vi "StaticCalibration.vi"(0 "SENSOR":T1, 11 "error in (no error)":errorcluster caption="错误输入（无错误）") -> (4 "Vres":dbl, 6 "Angle out":dbl, 8 "Vres_FD":i32, 10 "OK？":bool, 15 "error out":errorcluster caption="错误输出")   [LabVIEW 2020]
doc: "该模板用于创建子VI。"
uses:
  Global_Variable/Global.vi
panel:
  out "T2(%)":dbl
  out "T1(%)":dbl
  out "S(%)":dbl
  out "P(%)":dbl
  out "T2ROC_1+T2ROC_2":i32
  out "T1ROC_1+T1ROC_2":i32
  out "PROC_1":i32
  out "T2ROC_1":i32
  out "T1ROC_1":i32
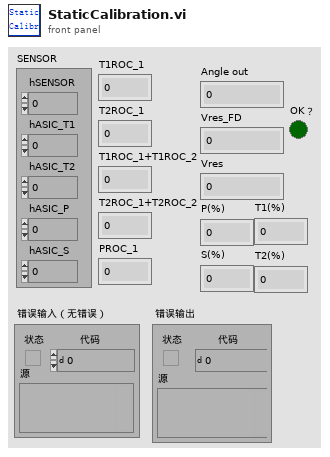
[diagram p1: front panel]
types:
  T1 = cluster{"hSENSOR":i32, "hASIC_T1":i32, "hASIC_T2":i32, "hASIC_P":i32, "hASIC_S":i32}
  T2 = cluster{"主信号":cluster{"单位":string, "下限":dbl, "上限":dbl}, "副信号":cluster{"单位":string, "下限":dbl, "上限":dbl}, "主副和":cluster{"单位":string, "下限":dbl, "上限":dbl}, "主副差":cluster{"单位":string, "下限":dbl, "上限":dbl}, "Vres":cluster{"单位":string, "下限":dbl, "上限":dbl}}
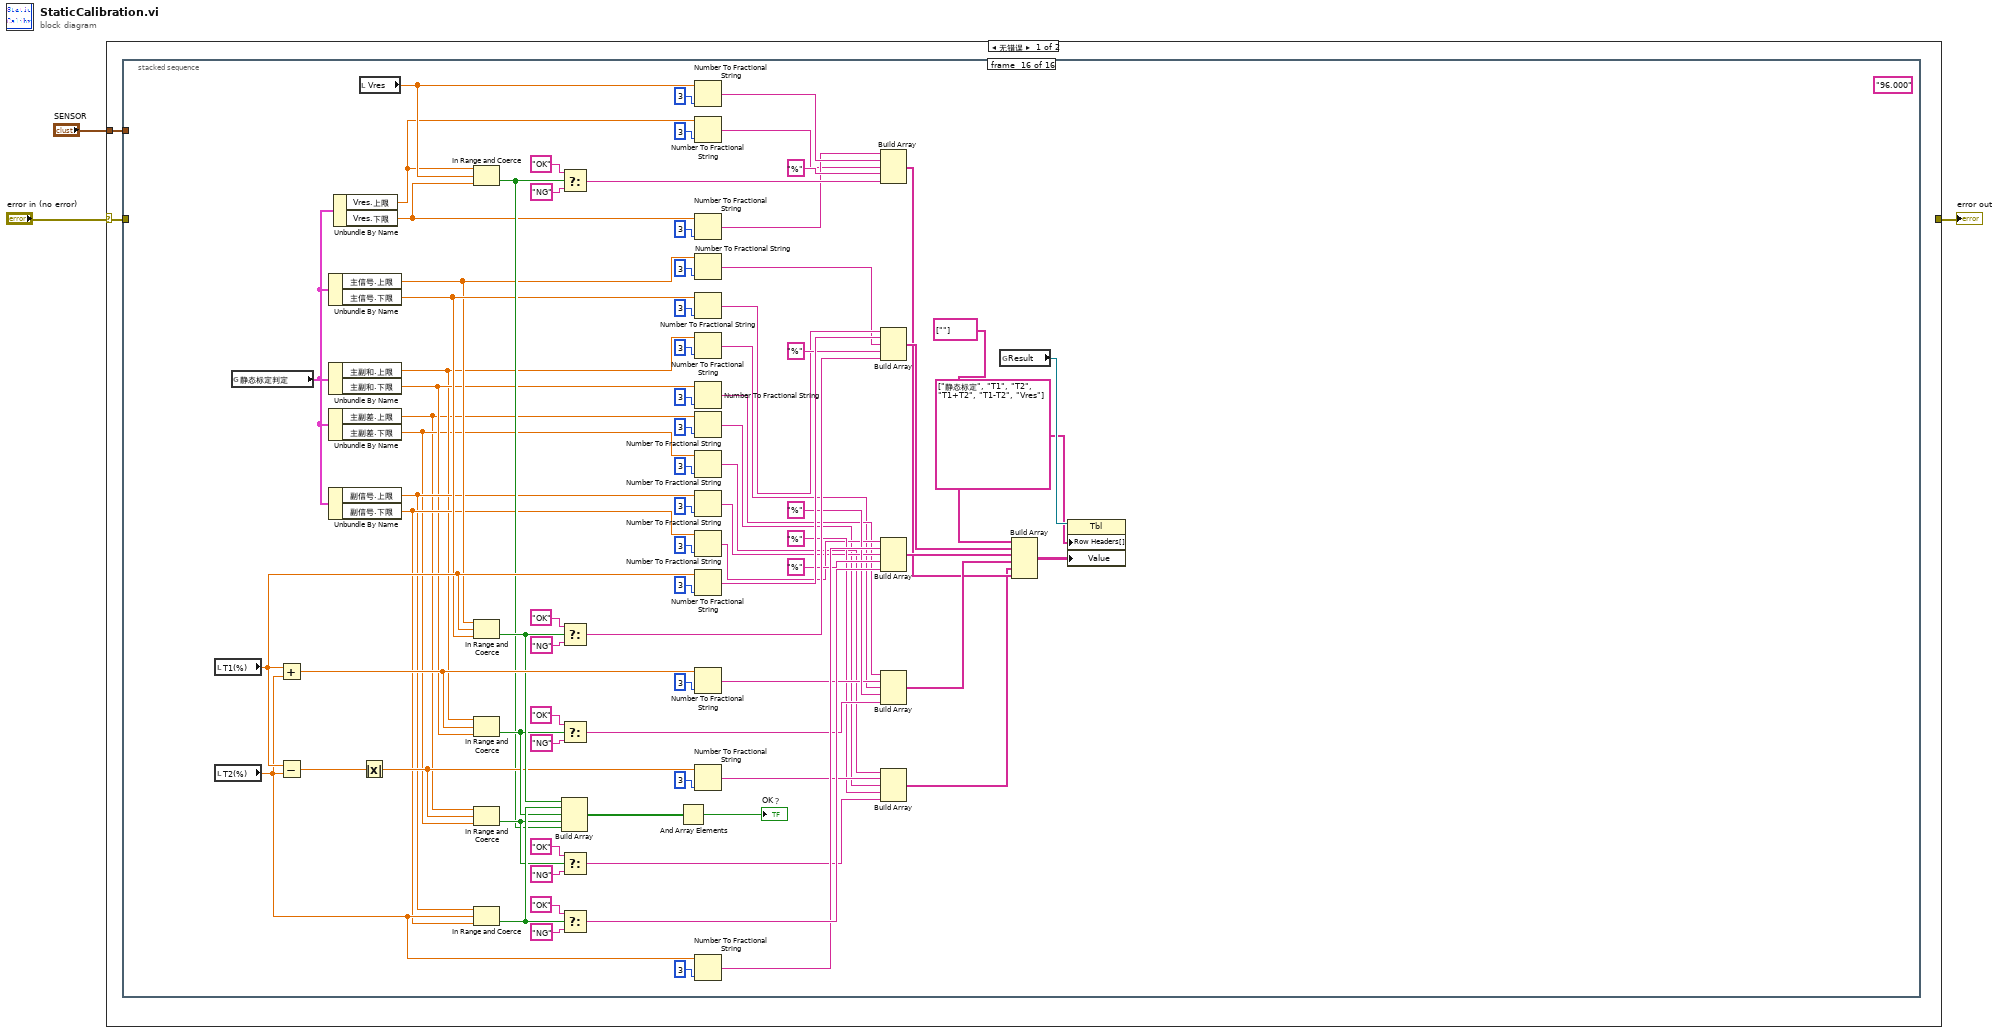
[diagram p0: block diagram]
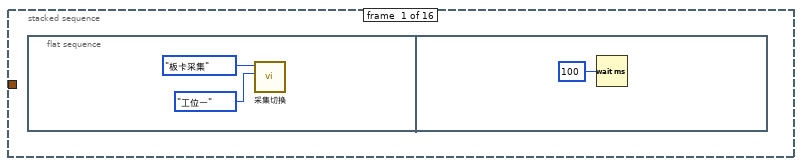
[diagram p2: hidden frame]
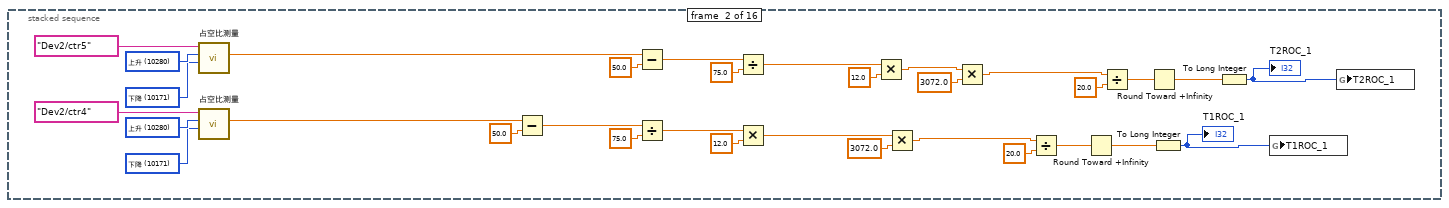
[diagram p3: hidden frame]
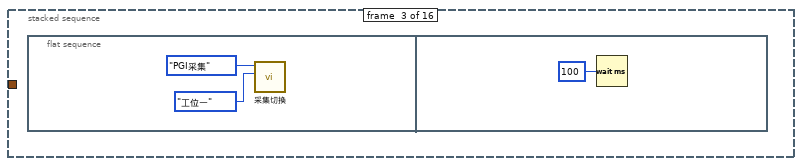
[diagram p4: hidden frame]
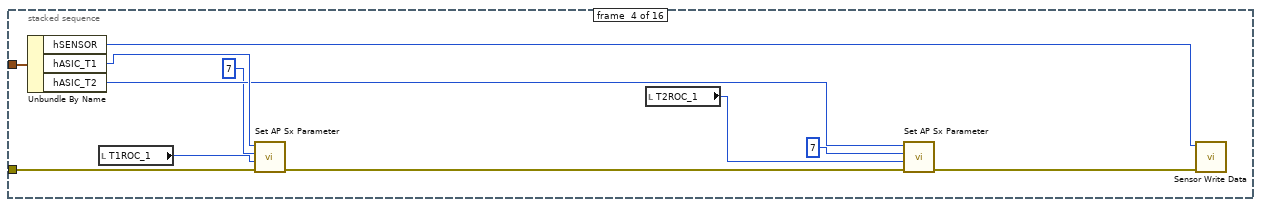
[diagram p5: hidden frame]
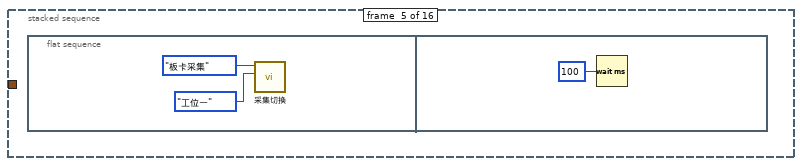
[diagram p6: hidden frame]
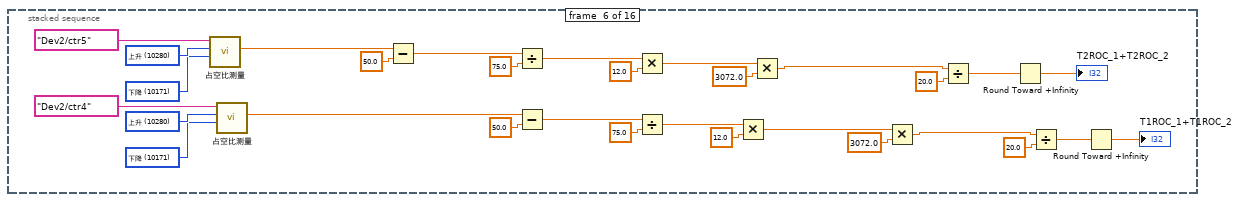
[diagram p7: hidden frame]
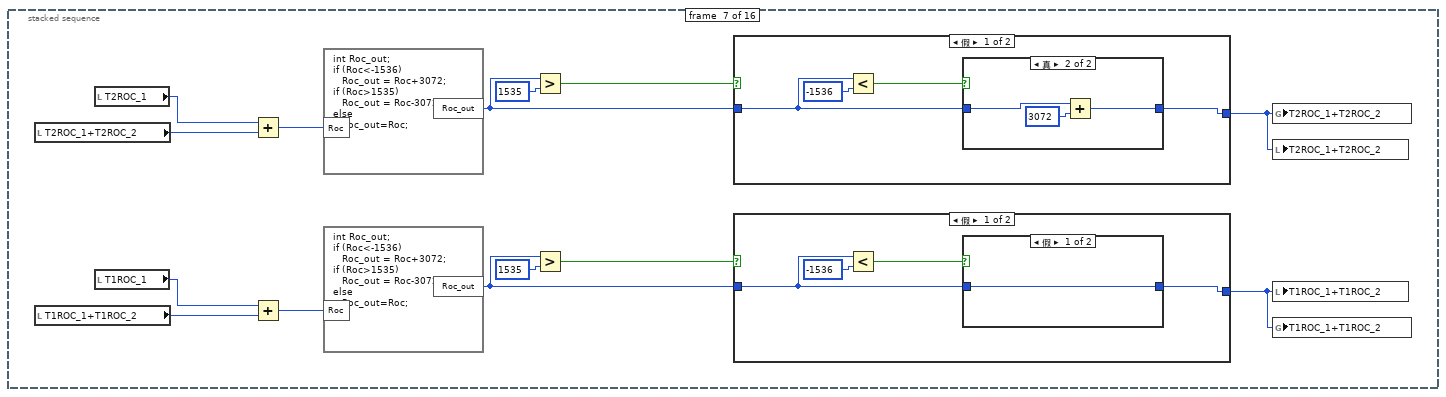
[diagram p8: hidden frame]
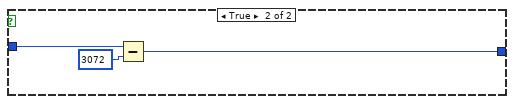
[diagram p10: hidden frame]
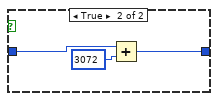
[diagram p11: hidden frame]
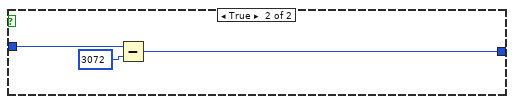
[diagram p12: hidden frame]
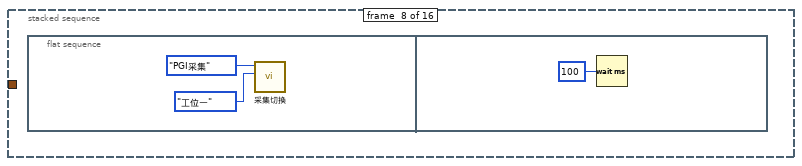
[diagram p13: hidden frame]
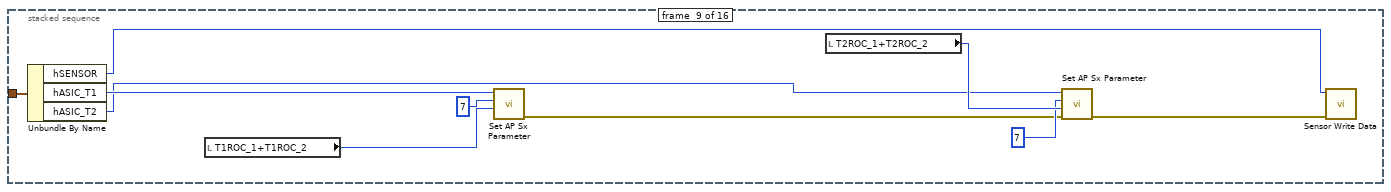
[diagram p14: hidden frame]
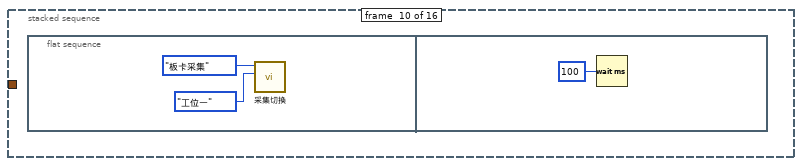
[diagram p15: hidden frame]
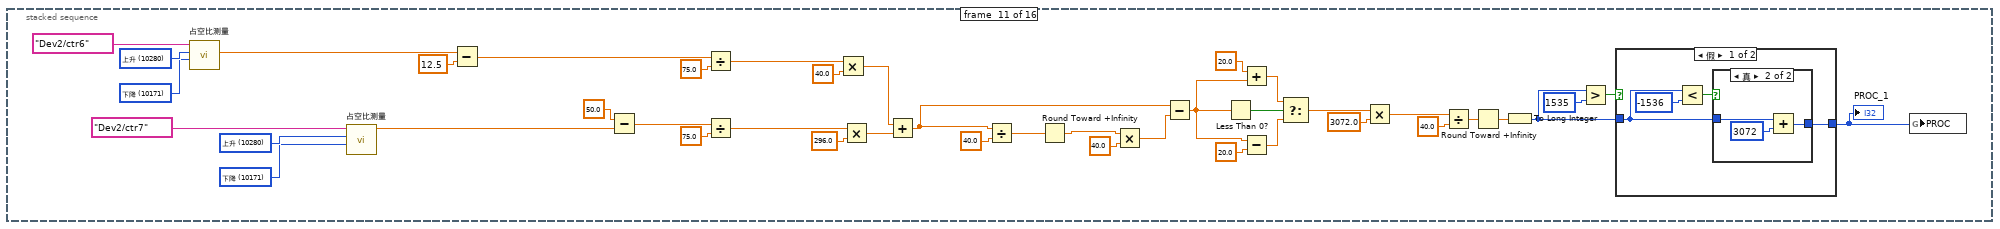
[diagram p16: hidden frame]
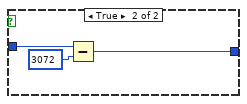
[diagram p18: hidden frame]
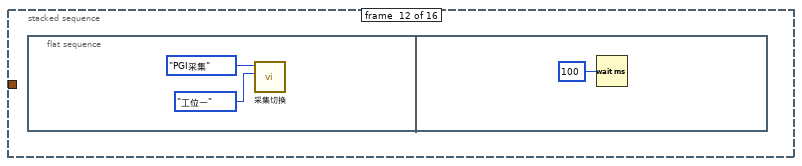
[diagram p19: hidden frame]
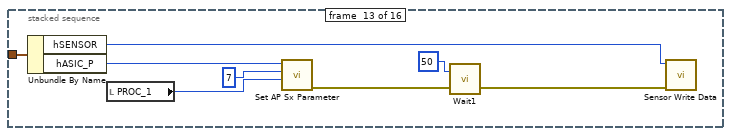
[diagram p20: hidden frame]
diagram:
  n1 = case shown="无错误" "error in (no error)" {
    selector: "error in (no error)" -> [w4 w309]
    tunnel: [_ w309] -> w2
    tunnel: "SENSOR" -> [w5 _]
    frame No Error {
      n2 = stacked-sequence {
        tunnel: w5 -> [_ _ _ w52 _ _ _ _ w135 _ _ _ w198 _ _ _]
        tunnel: w4 -> [_ _ _ w44 _ _ _ _ _ _ _ _ _ _ _ _]
        frame #0 {
          n3 = flat-sequence {
            frame #0 {
              n4 = call "采集切换.vi"("工位"=enum16{"工位一", "工位二"}."工位一", "采集方式"=enum16{"板卡采集", "PGI采集"}."板卡采集") -> ()  [unwired: 10 in]
            }
            frame #1 {
              n5 = Wait (ms)(milliseconds to wait=u32 100 ("等待时间（毫秒）")) -> ()  [unwired: 1 out]
            }
          }
        }
        frame #1 {
          w9 = 10171 items=["上升"=10280, "下降"=10171] ("starting edge2")
          w10 = 10280 items=["上升"=10280, "下降"=10171] ("starting edge1")
          w11 = 10171 items=["上升"=10280, "下降"=10171] ("starting edge2")
          w12 = 10280 items=["上升"=10280, "下降"=10171] ("starting edge1")
          n6 = call "占空比测量.vi"("计数器"=tag "Dev2/ctr5" ("counter"), "starting edge1"=w10, "starting edge2"=w9) -> ("占空比2(%)"=w13:dbl)  [unwired: 4 in, 3 out]
          n7 = call "占空比测量.vi"("计数器"=tag "Dev2/ctr4" ("counter"), "starting edge1"=w12, "starting edge2"=w11) -> ("占空比2(%)"=w16:dbl)  [unwired: 4 in, 3 out]
          n8 = Subtract(x=w16, y=50.0) -> (x-y=w39:dbl)
          n9 = Subtract(x=w13, y=50.0) -> (x-y=w24:dbl)
          n10 = Divide(x=w39, y=75.0) -> (x/y=w37:dbl)
          n11 = Divide(x=w24, y=75.0) -> (x/y=w26:dbl)
          n12 = Multiply(x=w37, y=12.0) -> (x*y=w35:dbl)
          n13 = Multiply(x=w26, y=12.0) -> (x*y=w28:dbl)
          n14 = Multiply(x=w35, y=3072.0) -> (x*y=w33:dbl)
          n15 = Multiply(x=w28, y=3072.0) -> (x*y=w30:dbl)
          n16 = Divide(x=w33, y=20.0) -> (x/y=w20:dbl)
          n17 = Round Toward +Infinity(x=w20) -> (ceil(x): smallest int >= x=w18:dbl)
          n18 = Divide(x=w30, y=20.0) -> (x/y=w19:dbl)
          n19 = Round Toward +Infinity(x=w19) -> (ceil(x): smallest int >= x=w17:dbl)
          n20 = To Long Integer(number=w18) -> (32bit integer=w14:i32)
          "T1ROC_1" <- w14
          n21 = To Long Integer(number=w17) -> (32bit integer=w15:i32)
          "T2ROC_1" <- w15
          n22 = global write "Global.vi" "T1ROC_1"(w14) -> ()
          n23 = global write "Global.vi" "T2ROC_1"(w15) -> ()
        }
        frame #2 {
          n24 = flat-sequence {
            frame #0 {
              n25 = call "采集切换.vi"("工位"=enum16{"工位一", "工位二"}."工位一", "采集方式"=enum16{"板卡采集", "PGI采集"}."PGI采集") -> ()  [unwired: 10 in]
            }
            frame #1 {
              n26 = Wait (ms)(milliseconds to wait=u32 100 ("等待时间（毫秒）")) -> ()  [unwired: 1 out]
            }
          }
        }
        frame #3 {
          n27 = Unbundle By Name(w52) -> ("hSENSOR"=w49:i32, "hASIC_T1"=w51:i32, "hASIC_T2"=w50:i32)
          n28 = local read "T1ROC_1"() -> (w53:i32)
          n29 = call "Set AP Sx Parameter.vi"("error in (no error)"=w44, "para2"=w53, "asicBitsName"=7, "asicHandle"=w51) -> ("error out"=w46:errorcluster)  [unwired: 6 in, 1 out]
          n30 = local read "T2ROC_1"() -> (w54:i32)
          n31 = call "Set AP Sx Parameter.vi"("error in (no error)"=w46, "para2"=w54, "asicBitsName"=7, "asicHandle"=w50) -> ("error out"=w45:errorcluster)  [unwired: 6 in, 1 out]
          n32 = call "Sensor Write Data.vi"("error in (no error)"=w45, "sensorHandle"=w49) -> ()  [unwired: 8 in, 2 out]
        }
        frame #4 {
          n33 = flat-sequence {
            frame #0 {
              n34 = call "采集切换.vi"("工位"=enum16{"工位一", "工位二"}."工位一", "采集方式"=enum16{"板卡采集", "PGI采集"}."板卡采集") -> ()  [unwired: 10 in]
            }
            frame #1 {
              n35 = Wait (ms)(milliseconds to wait=u32 100 ("等待时间（毫秒）")) -> ()  [unwired: 1 out]
            }
          }
        }
        frame #5 {
          w58 = 10171 items=["上升"=10280, "下降"=10171] ("starting edge2")
          w59 = 10280 items=["上升"=10280, "下降"=10171] ("starting edge1")
          w60 = 10171 items=["上升"=10280, "下降"=10171] ("starting edge2")
          w61 = 10280 items=["上升"=10280, "下降"=10171] ("starting edge1")
          n36 = call "占空比测量.vi"("计数器"=tag "Dev2/ctr5", "starting edge1"=w59, "starting edge2"=w58) -> ("占空比2(%)"=w65:dbl)  [unwired: 4 in, 3 out]
          n37 = call "占空比测量.vi"("计数器"=tag "Dev2/ctr4", "starting edge1"=w61, "starting edge2"=w60) -> ("占空比2(%)"=w62:dbl)  [unwired: 4 in, 3 out]
          n38 = Subtract(x=w65, y=50.0) -> (x-y=w87:dbl)
          n39 = Divide(x=w87, y=75.0) -> (x/y=w86:dbl)
          n40 = Subtract(x=w62, y=50.0) -> (x-y=w80:dbl)
          n41 = Multiply(x=w86, y=12.0) -> (x*y=w85:dbl)
          n42 = Divide(x=w80, y=75.0) -> (x/y=w81:dbl)
          n43 = Multiply(x=w81, y=12.0) -> (x*y=w82:dbl)
          n44 = Multiply(x=w85, y=3072.0) -> (x*y=w84:dbl)
          n45 = Multiply(x=w82, y=3072.0) -> (x*y=w83:dbl)
          n46 = Divide(x=w84, y=20.0) -> (x/y=w78:dbl)
          n47 = Round Toward +Infinity(x=w78) -> (ceil(x): smallest int >= x=→"T2ROC_1+T2ROC_2":dbl)
          n48 = Divide(x=w83, y=20.0) -> (x/y=w79:dbl)
          n49 = Round Toward +Infinity(x=w79) -> (ceil(x): smallest int >= x=→"T1ROC_1+T1ROC_2":dbl)
        }
        frame #6 {
          n50 = local read "T2ROC_1+T2ROC_2"() -> (w90:i32)
          n51 = local read "T1ROC_1+T1ROC_2"() -> (w91:i32)
          n52 = local read "T2ROC_1"() -> (w98:i32)
          n53 = local read "T1ROC_1"() -> (w99:i32)
          n54 = Add(x=w98, y=w90) -> (x+y=w100:i32)
          n55 = Add(x=w99, y=w91) -> (x+y=w101:i32)
          n56 = formula code="int Roc_out;\nif (Roc<-1536)\n   Roc_out = Roc+3072;\nif (Roc>1535)\n   Roc_out = Roc-3072;\nelse\n   Roc_out=Roc;"("Roc"=w100) -> ("Roc_out"=w92:i32)
          n57 = formula code="int Roc_out;\nif (Roc<-1536)\n   Roc_out = Roc+3072;\nif (Roc>1535)\n   Roc_out = Roc-3072;\nelse\n   Roc_out=Roc;"("Roc"=w101) -> ("Roc_out"=w95:i32)
          n58 = Greater?(x=w92, y=1535) -> (0:w93:bool)
          n59 = Greater?(x=w95, y=1535) -> (0:w96:bool)
          n60 = case shown="假" w93 {
            tunnel: w92 -> [w103 w111]
            tunnel: [w102 w110] -> w88
            frame False {
              n61 = Less?(x=w103, y=-1536) -> (x < y?=w104:bool)
              n62 = case shown="真" w104 {
                tunnel: w103 -> [w106 w109]
                tunnel: [w106 w107] -> w102
                frame False {
                }
                frame True {
                  n63 = Add(x=w109, y=3072) -> (x+y=w107:i32)
                }
              }
            }
            frame True {
              n64 = Subtract(x=w111, y=3072) -> (x-y=w110:i32)
            }
          }
          n65 = case shown="假" w96 {
            tunnel: w95 -> [w114 w122]
            tunnel: [w113 w121] -> w89
            frame False {
              n66 = Less?(x=w114, y=-1536) -> (x < y?=w115:bool)
              n67 = case shown="假" w115 {
                tunnel: w114 -> [w117 w120]
                tunnel: [w117 w118] -> w113
                frame False {
                }
                frame True {
                  n68 = Add(x=w120, y=3072) -> (x+y=w118:i32)
                }
              }
            }
            frame True {
              n69 = Subtract(x=w122, y=3072) -> (x-y=w121:i32)
            }
          }
          n70 = global write "Global.vi" "T2ROC_1+T2ROC_2"(w88) -> ()
          n71 = local write "T2ROC_1+T2ROC_2"(w88) -> ()
          n72 = local write "T1ROC_1+T1ROC_2"(w89) -> ()
          n73 = global write "Global.vi" "T1ROC_1+T1ROC_2"(w89) -> ()
        }
        frame #7 {
          n74 = flat-sequence {
            frame #0 {
              n75 = call "采集切换.vi"("工位"=enum16{"工位一", "工位二"}."工位一", "采集方式"=enum16{"板卡采集", "PGI采集"}."PGI采集") -> ()  [unwired: 10 in]
            }
            frame #1 {
              n76 = Wait (ms)(milliseconds to wait=u32 100 ("等待时间（毫秒）")) -> ()  [unwired: 1 out]
            }
          }
        }
        frame #8 {
          n77 = Unbundle By Name(w135) -> ("hSENSOR"=w132:i32, "hASIC_T1"=w134:i32, "hASIC_T2"=w133:i32)
          n78 = local read "T1ROC_1+T1ROC_2"() -> (w131:i32)
          n79 = call "Set AP Sx Parameter.vi"("para2"=w131, "asicBitsName"=7, "asicHandle"=w134) -> ("error out"=w128:errorcluster)  [unwired: 7 in, 1 out]
          n80 = local read "T2ROC_1+T2ROC_2"() -> (w136:i32)
          n81 = call "Set AP Sx Parameter.vi"("error in (no error)"=w128, "para2"=w136, "asicBitsName"=7, "asicHandle"=w133) -> ("error out"=w127:errorcluster)  [unwired: 6 in, 1 out]
          n82 = call "Sensor Write Data.vi"("error in (no error)"=w127, "sensorHandle"=w132) -> ()  [unwired: 8 in, 2 out]
        }
        frame #9 {
          n83 = flat-sequence {
            frame #0 {
              n84 = call "采集切换.vi"("工位"=enum16{"工位一", "工位二"}."工位一", "采集方式"=enum16{"板卡采集", "PGI采集"}."板卡采集") -> ()  [unwired: 10 in]
            }
            frame #1 {
              n85 = Wait (ms)(milliseconds to wait=u32 100 ("等待时间（毫秒）")) -> ()  [unwired: 1 out]
            }
          }
        }
        frame #10 {
          w140 = 10171 items=["上升"=10280, "下降"=10171] ("starting edge2")
          w141 = 10280 items=["上升"=10280, "下降"=10171] ("starting edge1")
          w142 = 10171 items=["上升"=10280, "下降"=10171] ("starting edge2")
          w143 = 10280 items=["上升"=10280, "下降"=10171] ("starting edge1")
          n86 = call "占空比测量.vi"("计数器"=tag "Dev2/ctr6", "starting edge1"=w143, "starting edge2"=w142) -> ("占空比2(%)"=w148:dbl)  [unwired: 4 in, 3 out]
          n87 = call "占空比测量.vi"("计数器"=tag "Dev2/ctr7", "starting edge1"=w141, "starting edge2"=w140) -> ("占空比(%)"=w147:dbl)  [unwired: 4 in, 3 out]
          n88 = Subtract(x=w148, y=12.5) -> (x-y=w180:dbl)
          n89 = Subtract(x=50.0, y=w147) -> (x-y=w174:dbl)
          n90 = Divide(x=w180, y=75.0) -> (x/y=w178:dbl)
          n91 = Divide(x=w174, y=75.0) -> (x/y=w172:dbl)
          n92 = Multiply(x=w178, y=40.0) -> (x*y=w176:dbl)
          n93 = Multiply(x=w172, y=296.0) -> (x*y=w170:dbl)
          n94 = Add(x=w176, y=w170) -> (x+y=w164:dbl)
          n95 = Divide(x=w164, y=40.0) -> (x/y=w168:dbl)
          n96 = Round Toward +Infinity(x=w168) -> (ceil(x): smallest int >= x=w166:dbl)
          n97 = Multiply(x=w166, y=40.0) -> (x*y=w165:dbl)
          n98 = Subtract(x=w164, y=w165) -> (x-y=w160:dbl)
          n99 = Less Than 0?(x=w160) -> (x < 0?=w159:bool)
          n100 = Add(x=20.0, y=w160) -> (x+y=w162:dbl)
          n101 = Subtract(x=w160, y=20.0 ("x")) -> (x-y=w158:dbl)
          n102 = Select(t=w162, s=w159, f=w158) -> (s? t:f=w157:dbl)
          n103 = Multiply(x=w157, y=3072.0) -> (x*y=w155:dbl)
          n104 = Divide(x=w155, y=40.0) -> (x/y=w150:dbl)
          n105 = Round Toward +Infinity(x=w150) -> (ceil(x): smallest int >= x=w149:dbl)
          n106 = To Long Integer(number=w149) -> (32bit integer=w153:i32)
          n107 = Greater?(x=w153, y=1535) -> (0:w151:bool)
          n108 = case shown="假" w151 {
            tunnel: w153 -> [w183 w191]
            tunnel: [w182 w190] -> w144
            frame False {
              n109 = Less?(x=w183, y=-1536) -> (x < y?=w184:bool)
              n110 = case shown="真" w184 {
                tunnel: w183 -> [w186 w189]
                tunnel: [w186 w187] -> w182
                frame False {
                }
                frame True {
                  n111 = Add(x=w189, y=3072) -> (x+y=w187:i32)
                }
              }
            }
            frame True {
              n112 = Subtract(x=w191, y=3072) -> (x-y=w190:i32)
            }
          }
          "PROC_1" <- w144
          n113 = global write "Global.vi" "PROC"(w144) -> ()
        }
        frame #11 {
          n114 = flat-sequence {
            frame #0 {
              n115 = call "采集切换.vi"("工位"=enum16{"工位一", "工位二"}."工位一", "采集方式"=enum16{"板卡采集", "PGI采集"}."PGI采集") -> ()  [unwired: 10 in]
            }
            frame #1 {
              n116 = Wait (ms)(milliseconds to wait=u32 100 ("等待时间（毫秒）")) -> ()  [unwired: 1 out]
            }
          }
        }
        frame #12 {
          n117 = Unbundle By Name(w198) -> ("hSENSOR"=w197:i32, "hASIC_P"=w196:i32)
          n118 = local read "PROC_1"() -> (w201:i32)
          n119 = call "Set AP Sx Parameter.vi"("para2"=w201, "asicBitsName"=7, "asicHandle"=w196) -> ("error out"=w203:errorcluster)  [unwired: 7 in, 1 out]
          n120 = call "Wait1.vi"("error in (no error)"=w203, "Wait（150ms）"=u32 50) -> ("error out"=w202:errorcluster)  [unwired: 1 in]
          n121 = call "Sensor Write Data.vi"("error in (no error)"=w202, "sensorHandle"=w197) -> ()  [unwired: 8 in, 2 out]
        }
        frame #13 {
          n122 = flat-sequence {
            frame #0 {
              n123 = call "采集切换.vi"("工位"=enum16{"工位一", "工位二"}."工位一", "采集方式"=enum16{"板卡采集", "PGI采集"}."板卡采集") -> ()  [unwired: 10 in]
            }
            frame #1 {
              n124 = Wait (ms)(milliseconds to wait=u32 100 ("等待时间（毫秒）")) -> ()  [unwired: 1 out]
            }
          }
        }
        frame #14 {
          w207 = 10171 items=["上升"=10280, "下降"=10171] ("starting edge2")
          w208 = 10280 items=["上升"=10280, "下降"=10171] ("starting edge1")
          w209 = 10171 items=["上升"=10280, "下降"=10171] ("starting edge2")
          w210 = 10280 items=["上升"=10280, "下降"=10171] ("starting edge1")
          w211 = 10171 items=["上升"=10280, "下降"=10171] ("starting edge2")
          w212 = 10280 items=["上升"=10280, "下降"=10171] ("starting edge1")
          w213 = 10171 items=["上升"=10280, "下降"=10171] ("starting edge2")
          w214 = 10280 items=["上升"=10280, "下降"=10171] ("starting edge1")
          n125 = call "占空比测量.vi"("计数器"=tag "Dev2/ctr4", "starting edge1"=w210, "starting edge2"=w209) -> ("占空比2(%)"=→"T1(%)":dbl)  [unwired: 4 in, 3 out]
          n126 = call "占空比测量.vi"("计数器"=tag "Dev2/ctr6", "starting edge1"=w214, "starting edge2"=w213) -> ("占空比2(%)"=w223:dbl)  [unwired: 4 in, 3 out]
          "P(%)" <- w223
          n127 = call "占空比测量.vi"("计数器"=tag "Dev2/ctr5", "starting edge1"=w208, "starting edge2"=w207) -> ("占空比2(%)"=→"T2(%)":dbl)  [unwired: 4 in, 3 out]
          n128 = call "占空比测量.vi"("计数器"=tag "Dev2/ctr7", "starting edge1"=w212, "starting edge2"=w211) -> ("占空比(%)"=w222:dbl)  [unwired: 4 in, 3 out]
          "S(%)" <- w222
          n129 = call "Calc_Vres.vi"("S_Data in"=w222, "P_Data in"=w223) -> ("Vres_FD"=→"Vres_FD":i32, "Vres"=→"Vres":dbl, "Angle out"=→"Angle out":dbl)  [unwired: 7 in]
        }
        frame #15 {
          (unwired) "96.000"
          n130 = local read "T1(%)"() -> (w261:dbl)
          n131 = local read "T2(%)"() -> (w260:dbl)
          n132 = global read "Global.vi" "静态标定判定"() -> (w258:T2)
          n133 = Add(x=w261, y=w260) -> (x+y=w299:dbl)
          n134 = Subtract(x=w261, y=w260) -> (x-y=w264:dbl)
          n135 = Unbundle By Name(w258) -> ("主信号.上限"=w243:dbl, "主信号.下限"=w245:dbl)
          n136 = Unbundle By Name(w258) -> ("主副和.上限"=w236:dbl, "主副和.下限"=w237:dbl)
          n137 = Unbundle By Name(w258) -> ("主副差.上限"=w234:dbl, "主副差.下限"=w235:dbl)
          n138 = Unbundle By Name(w258) -> ("副信号.上限"=w240:dbl, "副信号.下限"=w241:dbl)
          n139 = Unbundle By Name(w258) -> ("Vres.上限"=w232:dbl, "Vres.下限"=w233:dbl)
          n140 = local read "Vres"() -> (w303:dbl)
          n141 = Absolute Value(x=w264) -> (abs(x)=w259:dbl)
          n142 = In Range and Coerce(upper limit=w232, x=w303, lower limit=w233) -> (In Range?=w256:bool)  [unwired: 1 out]
          n143 = In Range and Coerce(upper limit=w243, x=w261, lower limit=w245) -> (In Range?=w275:bool)  [unwired: 1 out]
          n144 = In Range and Coerce(upper limit=w236, x=w299, lower limit=w237) -> (In Range?=w273:bool)  [unwired: 1 out]
          n145 = In Range and Coerce(upper limit=w234, x=w259, lower limit=w235) -> (In Range?=w257:bool)  [unwired: 1 out]
          n146 = In Range and Coerce(upper limit=w240, x=w260, lower limit=w241) -> (In Range?=w274:bool)  [unwired: 1 out]
          n147 = Build Array(w275, w274, w273, w257, w256) -> (w272:bool[])
          n148 = Select(t="OK", s=w256, f="NG") -> (s? t:f=w285:string)
          n149 = Select(t="OK", s=w275, f="NG") -> (s? t:f=w296:string)
          n150 = Select(t="OK", s=w273, f="NG") -> (s? t:f=w287:string)
          n151 = Select(t="OK", s=w257, f="NG") -> (s? t:f=w268:string)
          n152 = Select(t="OK", s=w274, f="NG") -> (s? t:f=w295:string)
          n153 = And Array Elements(Boolean array=w272) -> (logical AND=→"OK？":bool)
          n154 = Number To Fractional String(number=w303, precision (6)=i16 3 ("精度(6)")) -> (F-format string=w282:string)  [unwired: 2 in]
          n155 = Number To Fractional String(number=w232, precision (6)=i16 3 ("精度(6)")) -> (F-format string=w226:string)  [unwired: 2 in]
          n156 = Number To Fractional String(number=w233, precision (6)=i16 3 ("精度(6)")) -> (F-format string=w227:string)  [unwired: 2 in]
          n157 = Number To Fractional String(number=w243, precision (6)=i16 3 ("精度(6)")) -> (F-format string=w242:string)  [unwired: 2 in]
          n158 = Number To Fractional String(number=w245, precision (6)=i16 3 ("精度(6)")) -> (F-format string=w244:string)  [unwired: 2 in]
          n159 = Number To Fractional String(number=w236, precision (6)=i16 3 ("精度(6)")) -> (F-format string=w230:string)  [unwired: 2 in]
          n160 = Number To Fractional String(number=w237, precision (6)=i16 3 ("精度(6)")) -> (F-format string=w231:string)  [unwired: 2 in]
          n161 = Number To Fractional String(number=w234, precision (6)=i16 3 ("精度(6)")) -> (F-format string=w228:string)  [unwired: 2 in]
          n162 = Number To Fractional String(number=w235, precision (6)=i16 3 ("精度(6)")) -> (F-format string=w229:string)  [unwired: 2 in]
          n163 = Number To Fractional String(number=w240, precision (6)=i16 3 ("精度(6)")) -> (F-format string=w238:string)  [unwired: 2 in]
          n164 = Number To Fractional String(number=w241, precision (6)=i16 3 ("精度(6)")) -> (F-format string=w239:string)  [unwired: 2 in]
          n165 = Number To Fractional String(number=w261, precision (6)=i16 3 ("精度(6)")) -> (F-format string=w298:string)  [unwired: 2 in]
          n166 = Number To Fractional String(number=w299, precision (6)=i16 3 ("精度(6)")) -> (F-format string=w286:string)  [unwired: 2 in]
          n167 = Number To Fractional String(number=w259, precision (6)=i16 3 ("精度(6)")) -> (F-format string=w269:string)  [unwired: 2 in]
          n168 = Number To Fractional String(number=w260, precision (6)=i16 3 ("精度(6)")) -> (F-format string=w292:string)  [unwired: 2 in]
          n169 = Build Array(w227, w282, w226, "%", w285) -> (w277:string[])
          n170 = Build Array(w244, w298, w242, "%", w296) -> (w280:string[])
          n171 = Build Array(w239, w292, w238, "%", w295) -> (w279:string[])
          n172 = Build Array(w231, w286, w230, "%", w287) -> (w278:string[])
          n173 = Build Array(w229, w269, w228, "%", w268) -> (w262:string[])
          n174 = global read "Global.vi" "Result"() -> (w308:refnum<vi>)
          n175 = Build Array(string[] [""] ("元素"), w280, w279, w278, w262, w277) -> (w276:string[][])
          n176 = property class="Tbl"(reference=w308, "Row Headers[]"=string[] ["静态标定", "T1", "T2", "T1+T2", "T1-T2", "Vres"] ("行首字符串[]"), "Value"=w276) -> ()  [unwired: 1 in, 2 out]
        }
      }
    }
    frame Error {
    }
  }
  "error out" <- w2
